vi "Prober_LoadUnload.vi"(8 "error in (no error)":errorcluster, 11 "ProbeStationControl in":refnum<class "ProbeStationControl.lvclass">) -> (0 "error out":errorcluster, 2 "Home or Load?":enum16{"Measure", "Load"}(ring), 3 "ProbeStationControl out":refnum<class "ProbeStationControl.lvclass">)   [LabVIEW 2019, in "ProbeStationControl.lvclass"]
uses:
  ProbeStationControl.lvclass
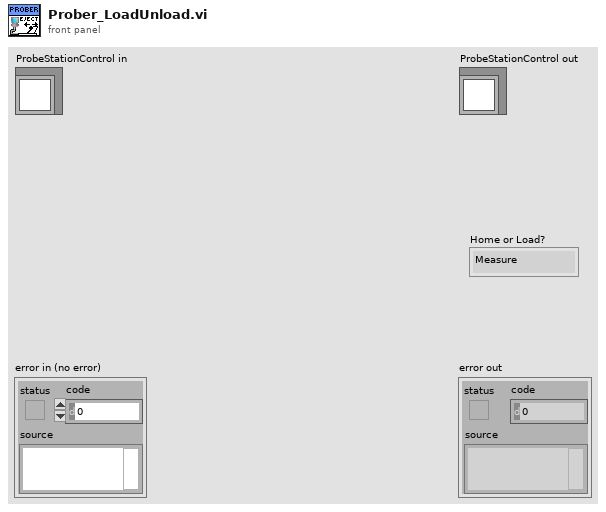
[diagram p1: front panel]
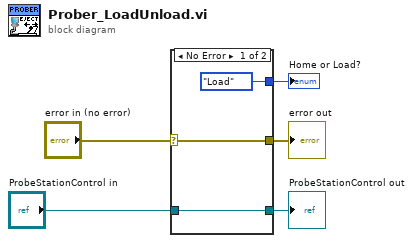
[diagram p0: block diagram]
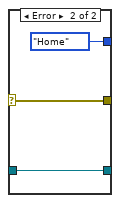
[diagram p2: hidden frame]
diagram:
  n1 = case shown="No Error" "error in (no error)" {
    selector: "error in (no error)" -> [w7 w11]
    tunnel: [w7 w11] -> w4
    tunnel: "ProbeStationControl in" -> [w8 w9]
    tunnel: [enum16{"Measure", "Load"}."Load" ("Home or Load?") enum16{"Home", "Load"}."Home" ("Home or Load?")] -> w3
    tunnel: [w8 w9] -> w1
    frame No Error {
    }
    frame Error {
    }
  }
  "error out" <- w4
  "Home or Load?" <- w3
  "ProbeStationControl out" <- w1
